vi "Postfix Traversal of Nodes.vi"(8 "error in (no error)":errorcluster, 11 "Generic in":refnum<vi>) -> (0 "error out":errorcluster, 3 "Array":T1[](array[typedef]))   [LabVIEW 2018, in "RPN.lvlib"]
uses:
  RPN.lvlib
  Node Type Def.ctl
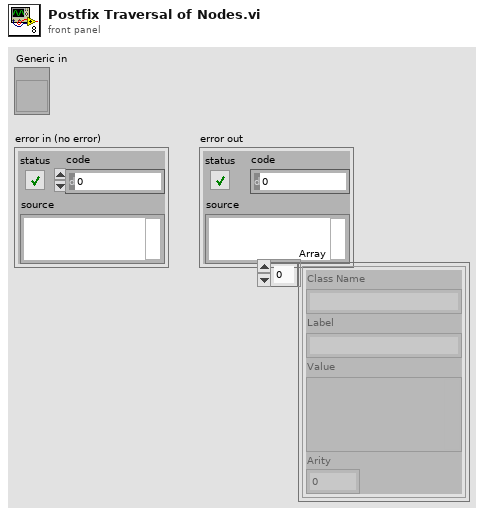
[diagram p1: front panel]
types:
  T1 = typedef "RPN.lvlib/Node Type Def.ctl" = cluster{"Class Name":string, "Label":string, "Value":variant, "Arity":u8}
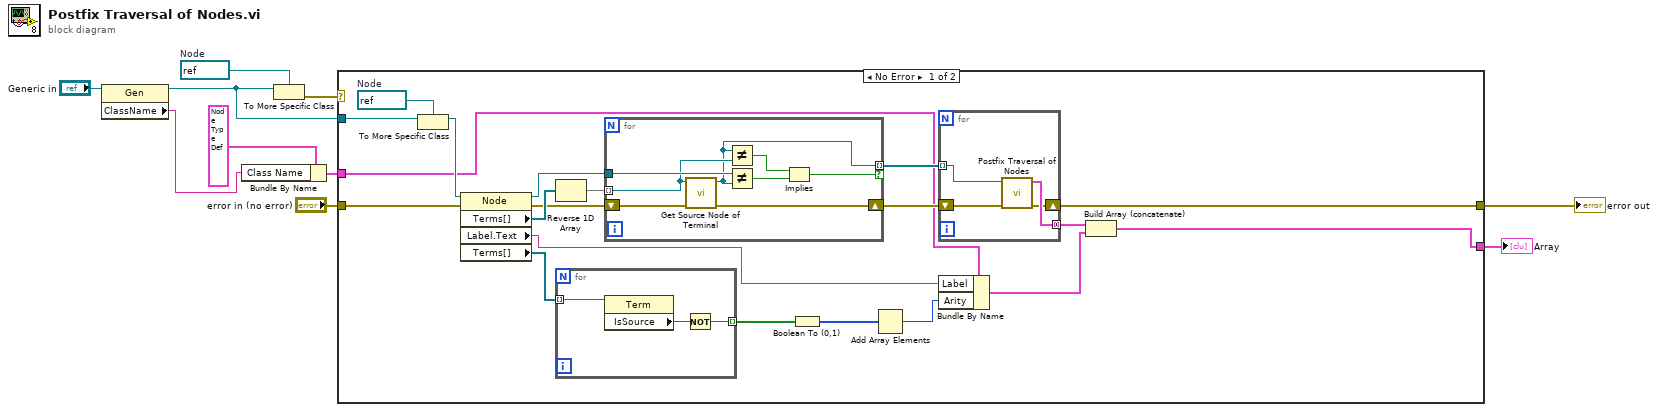
[diagram p0: block diagram]
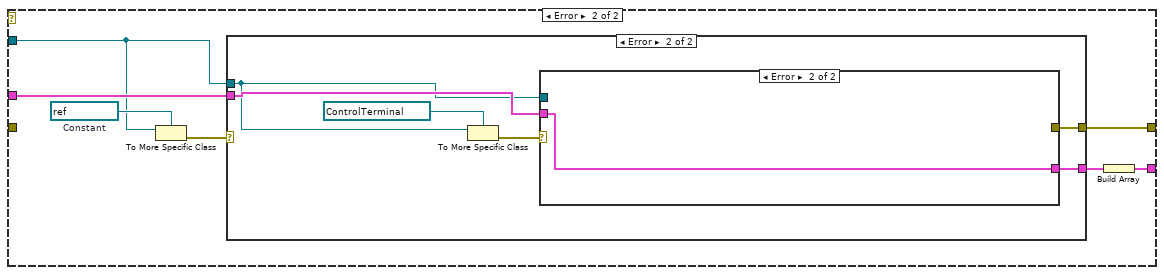
[diagram p2: hidden frame]
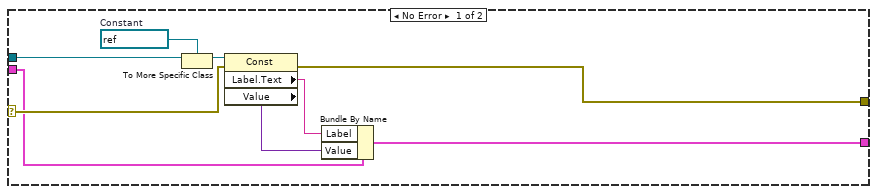
[diagram p3: hidden frame]
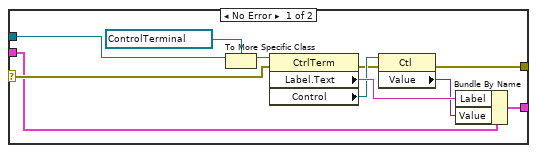
[diagram p4: hidden frame]
diagram:
  w7 = refnum<vi> refnum  # Node
  n1 = property class="Gen"(reference="Generic in") -> (reference out=w2:refnum<vi>, "ClassName"=w4:string)  [unwired: 1 in, 1 out]
  n2 = Bundle By Name(cluster=T1 {"Class Name"="", "Label"="", "Value"=variant, "Arity"=0}, "Class Name"=w4) -> (w5:T1)
  n3 = To More Specific Class(target class=w7, reference=w2) -> (error out=w8:errorcluster)  [unwired: 1 in, 1 out]
  n4 = case shown="No Error" w8 {
    tunnel: "error in (no error)" -> [w30 _]
    tunnel: [w22 w46] -> w10
    tunnel: [w25 w51] -> w1
    tunnel: w2 -> [w21 w47]
    tunnel: w5 -> [w18 w49]
    frame No Error {
      w19 = refnum<vi> refnum  # Node
      n5 = To More Specific Class(target class=w19, reference=w21) -> (specific class reference=w20:refnum<vi>)  [unwired: 1 in, 1 out]
      n6 = property class="Node"(reference=w20, error in=w30) -> (reference out=w28:refnum<vi>, error out=w24:errorcluster, "Terms[]"=w29:refnum<vi>[], "Label.Text"=w17:string, "Terms[]"=w14:refnum<vi>[])
      n7 = Reverse 1D Array(array=w29) -> (reversed array=w26:refnum<vi>[])
      n8 = for {
        tunnel: w14 -> [w33] mode=indexing
        tunnel: [w31] -> w13 mode=indexing
        n9 = property class="Term"(reference=w33) -> ("IsSource"=w32:bool)  [unwired: 1 in, 2 out]
        n10 = Not(x=w32) -> (.not. x?=w31:bool)
      }
      n11 = for {
        tunnel: w26 -> [w42] mode=indexing
        tunnel: w28 -> [w45]
        tunnel: [w41] -> w27 mode=indexing if=w38
        shift-right: [w43] -> w23
        shift-left: w24 -> [w44]
        n12 = call "Get Source Node of Terminal.vi"("error in (no error)"=w44, "Terminal in"=w42) -> ("error out"=w43:errorcluster, "Generic out"=w41:refnum<vi>)  [unwired: 8 in]
        n13 = Not Equal?(x=w41, y=w42) -> (x != y?=w40:bool)
        n14 = Not Equal?(x=w45, y=w41) -> (x != y?=w39:bool)
        n15 = Implies(1:w39, 2:w40) -> (0:w38:bool)
      }
      n16 = Boolean To (0,1)(Boolean=w13) -> (0, 1=w12:i16[])
      n17 = Add Array Elements(numeric array=w12) -> (sum=w11:i16)
      n18 = for {
        tunnel: w27 -> [w36] mode=indexing
        tunnel: [w37] -> w15 mode=concatenating
        shift-right: [w34] -> w22
        shift-left: w23 -> [w35]
        n19 = call "Postfix Traversal of Nodes.vi"("error in (no error)"=w35, "Generic in"=w36) -> ("error out"=w34:errorcluster, "Array"=w37:T1[])  [unwired: 8 in]
      }
      n20 = Bundle By Name(cluster=w18, "Label"=w17, "Arity"=w11) -> (w16:T1)
      n21 = Build Array (concatenate)(w15, w16) -> (w25:T1[])
    }
    frame Error {
      w52 = refnum<vi> refnum  # Constant
      n22 = To More Specific Class(target class=w52, reference=w47) -> (error out=w50:errorcluster)  [unwired: 1 in, 1 out]
      n23 = case shown="Error" w50 {
        selector: w50 -> [w61 _]
        tunnel: w49 -> [w60 w65]
        tunnel: [w58 w64] -> w48
        tunnel: w47 -> [w54 w63]
        tunnel: [w57 w66] -> w46
        frame No Error {
          w53 = refnum<vi> refnum  # Constant
          n24 = To More Specific Class(target class=w53, reference=w54) -> (specific class reference=w55:refnum<vi>)  [unwired: 1 in, 1 out]
          n25 = property class="Const"(reference=w55, error in=w61) -> (error out=w57:errorcluster, "Label.Text"=w56:string, "Value"=w59:variant)  [unwired: 1 out]
          n26 = Bundle By Name(cluster=w60, "Label"=w56, "Value"=w59) -> (w58:T1)
        }
        frame Error {
          n27 = To More Specific Class(target class=refnum<vi> refnum ("Terminal"), reference=w63) -> (error out=w67:errorcluster)  [unwired: 1 in, 1 out]
          n28 = case shown="Error" w67 {
            selector: w67 -> [w78 _]
            tunnel: [w69 _] -> w66
            tunnel: w65 -> [w68 w79]
            tunnel: [w77 w79] -> w64
            tunnel: w63 -> [w75 _]
            frame No Error {
              n29 = To More Specific Class(target class=refnum<vi> refnum ("Terminal"), reference=w75) -> (specific class reference=w74:refnum<vi>)  [unwired: 1 in, 1 out]
              n30 = property class="CtrlTerm"(reference=w74, error in=w78) -> (error out=w70:errorcluster, "Label.Text"=w76:string, "Control"=w72:refnum<vi>)  [unwired: 1 out]
              n31 = property class="Ctl"(reference=w72, error in=w70) -> (error out=w69:errorcluster, "Value"=w71:variant)  [unwired: 1 out]
              n32 = Bundle By Name(cluster=w68, "Label"=w76, "Value"=w71) -> (w77:T1)
            }
            frame Error {
            }
          }
        }
      }
      n33 = Build Array(w48) -> (w51:T1[])
    }
  }
  "error out" <- w10
  "Array" <- w1
